vi "CloseVLCPlayer.vi"(8 "error in":errorcluster, 11 "Connection ID in":refnum<k5>) -> (0 "error out":errorcluster)   [LabVIEW 2015]
doc: "Close the VLC player instance. This will send a quit signal to the VLC process and close the TCP connection."
uses:
  VLCCommand.ctl
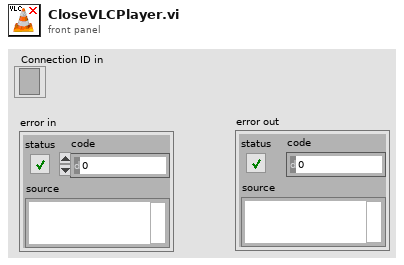
[diagram p1: front panel]
types:
  T1 = typedef "VLCCommand.ctl" = enum16{"add", "enqueue", "playlist", "play", "stop", "next", "prev", "goto", "repeat", "loop", "random", "clear", "status", "title", "title_n", "title_p", "chapter", "chapter_n", "chapter_p", "seek", "pause", "fastforward", "rewind", "faster", "slower", "normal", "frame", "f", "info", "stats", "get_time", "is_playing", "get_title", "get_length", "volume", "volup", "voldown", "adev", "achan", "atrack", "vtrack", "vratio", "vcrop", "vzoom", "snapshot", "strack", "key", "help", "logout", "quit"}
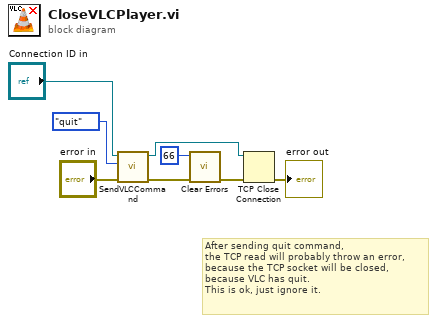
[diagram p0: block diagram]
diagram:
  # "After sending quit command, \nthe TCP read will probably throw an error, \nbecause the TCP socket will be closed, \nbecause VLC has quit.\nThis is ok, just ignore it."
  n1 = call "SendVLCCommand.vi"("error in"="error in", "Command"=VLCCommand."quit", "Connection ID in"="Connection ID in") -> ("error out"=w7:errorcluster, "Connection ID out"=w8:refnum<k5>)  [unwired: 5 in, 2 out]
  n2 = call <vilib>:"Clear Errors.vi"("error in (no error)"=w7, "specific error code to clear (0: all)"=66) -> ("error out"=w2:errorcluster)  [unwired: 4 in, 1 out]
  n3 = TCP Close Connection(connection ID=w8, error in (no error)=w2) -> (error out=→"error out":errorcluster)  [unwired: 1 in, 1 out]
